vi "Pre Launch Init.vi"(11 "Samples in":refnum<class "Samples.lvclass">) -> (0 "error out":errorcluster, 3 "Samples out":refnum<class "Samples.lvclass">)   [LabVIEW 2015, in "AMS UI.lvlib" / "Samples.lvclass"]
doc: "(<B>Filename</B>: Actor Framework.lvlib:Actor.lvclass:Pre Launch Init.vi)\n\nDefines behavior that occurs after the Launch Actor method is invoked but before the actor's Actor Core method begins running.\n\nThe Pre Launch Init method is guaranteed to finish before the Launch Actor method returns to its caller and before the actor itself receives any messages. Any references that the Pre Launch Init method obtains are guaranteed to have the same lifetime as the actor itself. Any errors that the Pre Launch Init method returns will abort the launch.\n\nBy default, this method does nothing. A descendant class may override it to define behavior."
uses:
  Samples.lvclass
  AMS Gas Actor/AMS Gas Actor.lvclass
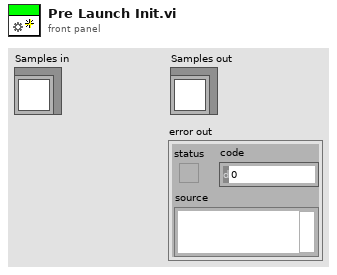
[diagram p1: front panel]
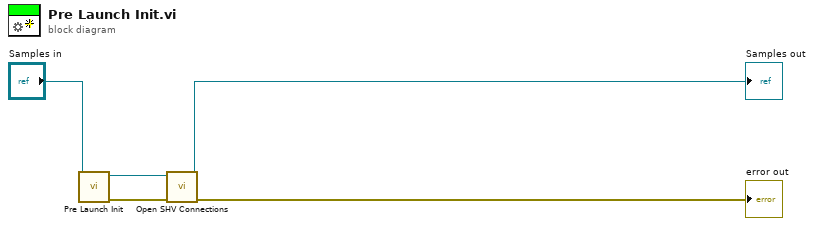
[diagram p0: block diagram]
diagram:
  n1 = call-parent "Pre Launch Init.vi"("eActor in"="Samples in") -> ("error out"=w5:errorcluster, "eActor out"=w3:refnum<class "Samples.lvclass">)  [unwired: 9 in]
  n2 = call "Open SHV Connections.vi"("error in (no error)"=w5, "Samples in"=w3) -> ("error out"=→"error out":errorcluster, "Samples out"=→"Samples out":refnum<class "Samples.lvclass">)  [unwired: 8 in]
